vi "gfitsio-get-column-info.vi"(6 "row (-1: don't check descriptor)":i32=-1, 7 "column":string, 8 "error in (no error)":errorcluster, 9 "case sensitive? (F:No)":bool, 11 "gfits refnum":T2) -> (0 "error out":errorcluster, 1 "variable length array?":bool, 2 "nelements":i32, 3 "dup gfits refnum":T2, 4 "column number":i32, 5 "cfitsio datatype":T1=1 items=["TBIT"=1, "TBYTE  (U8)"=11, "TSBYTE  (I8)"=12, "TLOGICAL"=14, "TSTRING"=16, "TUSHORT  (U16)"=20, "TSHORT  (I16)"=21, "TUINT"=31, "TULONG  (U32)"=40, "TLONG  (I32)"=41, "TFLOAT  (SGL)"=42, "TLONGLONG  (I64)"=81, "TDOUBLE  (DBL)"=82, "TCOMPLEX  (CSG)"=83, "TDOUBLECOMPLEX  (CDB)"=163])   [LabVIEW 2019, in "gfitsio.lvlib"]
doc: "Return the data type of a column in an ASCII or binary table. In the case of scaled integer columns it returns the 'equivalent' data type that is needed to store the scaled values, and not necessarily the physical data type of the unscaled values as stored in the FITS table. For example if a '1I' column in a binary table has TSCALn = 1 and TZEROn = 32768, then this column effectively contains unsigned short integer values, and thus the returned value of typecode will be TUSHORT, not TSHORT. Similarly, if a column has TTYPEn = '1I' and TSCALn = 0.12, then the returned typecode will be TFLOAT."
uses:
  gfitsio.lvlib
  gfitsio-refnum.ctl
  cfitsio-datatypes.ctl
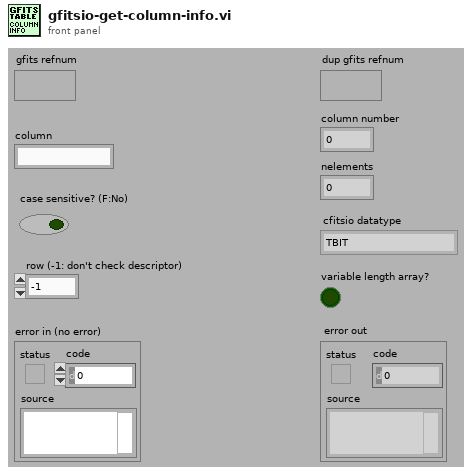
[diagram p1: front panel]
types:
  T1 = typedef "gfitsio.lvlib/cfitsio-datatypes.ctl" = i32
  T2 = typedef "gfitsio.lvlib/gfitsio-refnum.ctl" = refnum<k1>
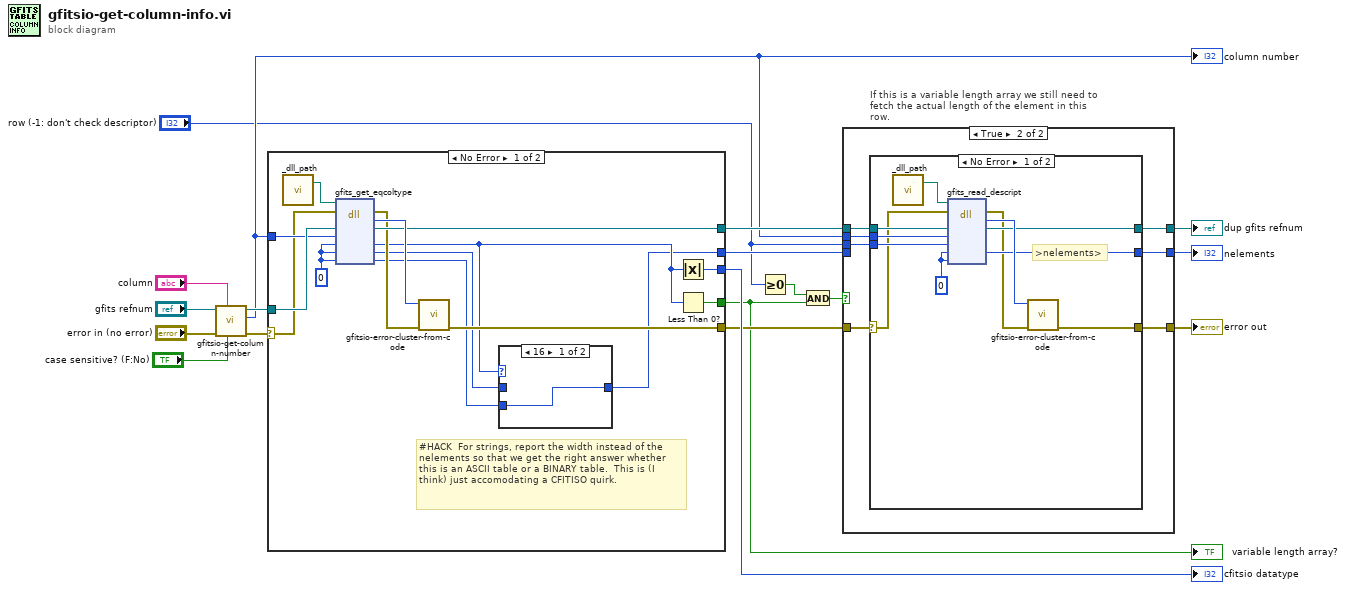
[diagram p0: block diagram]
diagram:
  n1 = call "gfitsio-get-column-number.vi"("case sensitive? (F:No)"="case sensitive? (F:No)", "column"="column", "error in (no error)"="error in (no error)", "gfits refnum"="gfits refnum") -> ("error out"=w15:errorcluster, "colnum"=w8:i32, "dup gfits refnum"=w13:T2)  [unwired: 5 in]
  "column number" <- w8
  n2 = case shown="No Error" w15 {
    selector: w15 -> [w26 w37]
    tunnel: [w32 w37] -> w11
    tunnel: w13 -> [w30 w36]
    tunnel: [w31 w36] -> w10
    tunnel: w8 -> [w29 _]
    tunnel: [w28 _] -> w18
    tunnel: [w27 _] -> w2
    tunnel: [w20 _] -> w6
    frame No Error {
      w24 = 0
      # "#HACK  For strings, report the width instead of the nelements so that we get the right answer whether this is an ASCII table or a BINARY table.  This is (I think) just accomodating a CFITISO quirk."
      n3 = call "_dll_path.vi"() -> ("Path"=w19:path)  [unwired: 1 in]
      n4 = dll-call lib="?" fn="gfits_get_eqcoltype"(path in=w19, error in=w26, "refnum"=w30, "colnum"=w29, "datatype"=w24, "nelements"=w24, "width"=w24) -> (error out=w25:errorcluster, "return type"=w33:i32, "refnum"=w31:T2, "datatype"=w23:i32, "nelements"=w21:i32, "width"=w22:i32)  [unwired: 2 in, 1 out]
      n5 = call "gfitsio-error-cluster-from-code.vi"("error in (no error)"=w25, "error code"=w33) -> ("error out"=w32:errorcluster)  [unwired: 9 in]
      n6 = case shown="16" w23 {
        tunnel: w21 -> [_ w35]
        tunnel: w22 -> [w34 _]
        tunnel: [w34 w35] -> w20
        frame 16 {
        }
        frame Default {
        }
      }
      n7 = Absolute Value(x=w23) -> (abs(x)=w28:i32)
      n8 = Less Than 0?(x=w23) -> (x < 0?=w27:bool)
    }
    frame Error {
    }
  }
  "cfitsio datatype" <- w18
  "variable length array?" <- w2
  n9 = Greater Or Equal To 0?(x="row (-1: don't check descriptor)") -> (x >= 0?=w4:bool)
  n10 = And(x=w4, y=w2) -> (x .and. y?=w3:bool)
  n11 = case "If this is a variable length array we still need to fetch the actual length of the element in this row." shown="True" w3 {
    tunnel: [w38 w47] -> w1
    tunnel: [w39 w46] -> w9
    tunnel: [w40 w45] -> w7
    tunnel: "row (-1: don't check descriptor)" -> [_ w44]
    tunnel: w11 -> [w38 w43]
    tunnel: w10 -> [w39 w42]
    tunnel: w8 -> [_ w41]
    tunnel: w6 -> [w40 _]
    frame False {
      # ">nelements>"
    }
    frame True {
      n12 = case shown="No Error" w43 {
        selector: w43 -> [w50 w60]
        tunnel: [w57 w60] -> w47
        tunnel: w42 -> [w55 w59]
        tunnel: [w56 w59] -> w46
        tunnel: [w51 _] -> w45
        tunnel: w41 -> [w54 _]
        tunnel: w44 -> [w52 _]
        frame No Error {
          w53 = 0
          # ">nelements>"
          n13 = call "_dll_path.vi"() -> ("Path"=w48:path)  [unwired: 1 in]
          n14 = dll-call lib="?" fn="gfits_read_descript"(path in=w48, error in=w50, "refnum"=w55, "colnum"=w54, "row"=w52, "nelements"=w53, "offset"=w53) -> (error out=w49:errorcluster, "return type"=w58:i32, "refnum"=w56:T2, "nelements"=w51:i32)  [unwired: 3 in, 2 out]
          n15 = call "gfitsio-error-cluster-from-code.vi"("error in (no error)"=w49, "error code"=w58) -> ("error out"=w57:errorcluster)  [unwired: 9 out]
        }
        frame Error {
        }
      }
    }
  }
  "error out" <- w1
  "dup gfits refnum" <- w9
  "nelements" <- w7
